vi "Serial_WriteRead.vi"(8 "error in (no error)":errorcluster, 9 "Code":string, 10 "Console In":string, 11 "Python":T1) -> (0 "error out":errorcluster, 2 "Console":string, 3 "Python":T1)   [LabVIEW 2020]
uses:
  PythonCtrl.ctl
panel:
  out "replies":string[](array[string])
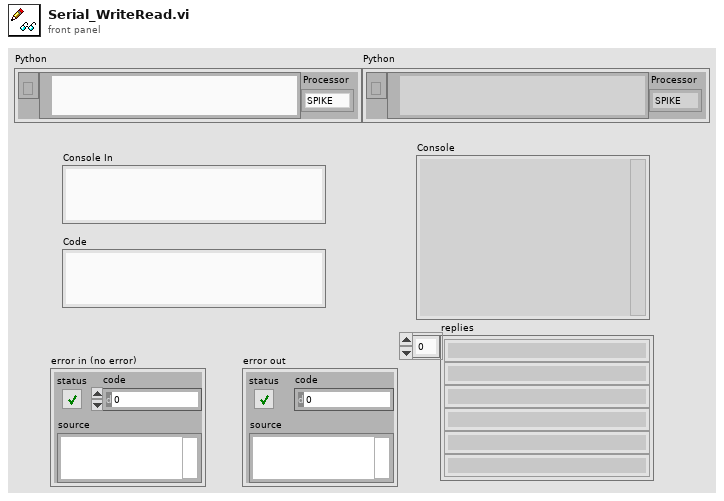
[diagram p1: front panel]
types:
  T1 = typedef "PythonCtrl.ctl" = cluster{"session":refnum<k35>, "PyPath":path, "Processor":enum16{"SPIKE", "Pi"}}
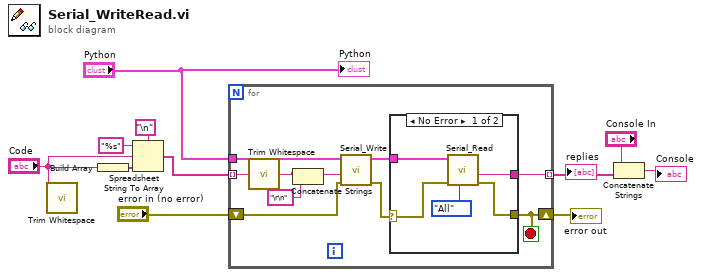
[diagram p0: block diagram]
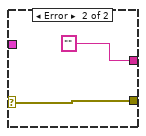
[diagram p2: hidden frame]
diagram:
  n1 = call <vilib>:"Trim Whitespace.vi"("string"="Code") -> ()  [unwired: 1 in, 1 out]
  n2 = Build Array("Code") -> (w6:string[])
  n3 = Spreadsheet String To Array(delimiter (Tab)="\n", format string="%s", spreadsheet string="Code", array type (2D Dbl)=w6) -> (array=w3:string[])
  n4 = for {
    tunnel: "Python" -> [w18]
    tunnel: w3 -> [w15] mode=indexing
    tunnel: [w17] -> w8 mode=indexing
    shift-right: [w16] -> w10
    shift-left: "error in (no error)" -> [w20]
    stop <- w16 stop-if-true
    n5 = call <vilib>:"Trim Whitespace.vi"("string"=w15) -> ("trimmed string"=w13:string)  [unwired: 1 in]
    n6 = Concatenate Strings(w13, "\r\n" ("delimiter (Tab)")) -> (w14:string)
    n7 = call "Serial_Write.vi"("error in (no error)"=w20, "Text to write"=w14, "Python"=w18) -> ("error out"=w19:errorcluster)  [unwired: 8 in]
    n8 = case shown="No Error" w19 {
      selector: w19 -> [w21 w26]
      tunnel: [w25 w26] -> w16
      tunnel: [w22 ""] -> w17
      tunnel: w18 -> [w24 _]
      frame No Error {
        n9 = call "Serial_Read.vi"("Task"=enum16{"Instant", "All"}."All", "error in (no error)"=w21, "Python"=w24) -> ("error out"=w25:errorcluster, "Text read"=w22:string)  [unwired: 7 in]
      }
      frame Error {
      }
    }
  }
  "error out" <- w10
  "replies" <- w8
  n10 = Concatenate Strings("Console In", w8) -> (→"Console":string)
  "Python" <- "Python"
